vi "loim.vi"() -> ()   [LabVIEW 2015]
panel:
  out "Játékos neve:":string
  out "Nyereménye:":string
  out "Nyereménylista:":i32(listbox)
  out "D válasz":string
  out "C válasz":string
  out "B válasz":string
  out "A válasz":string
  out "Kérdés":string
  in  "Kilépés":bool
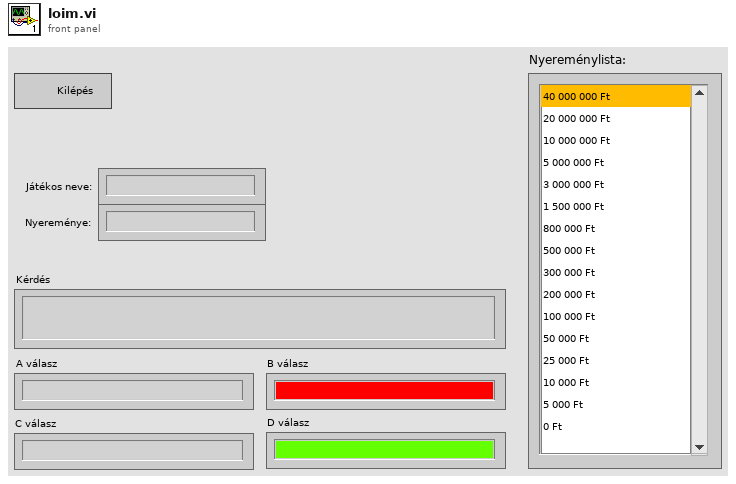
[diagram p1: front panel]
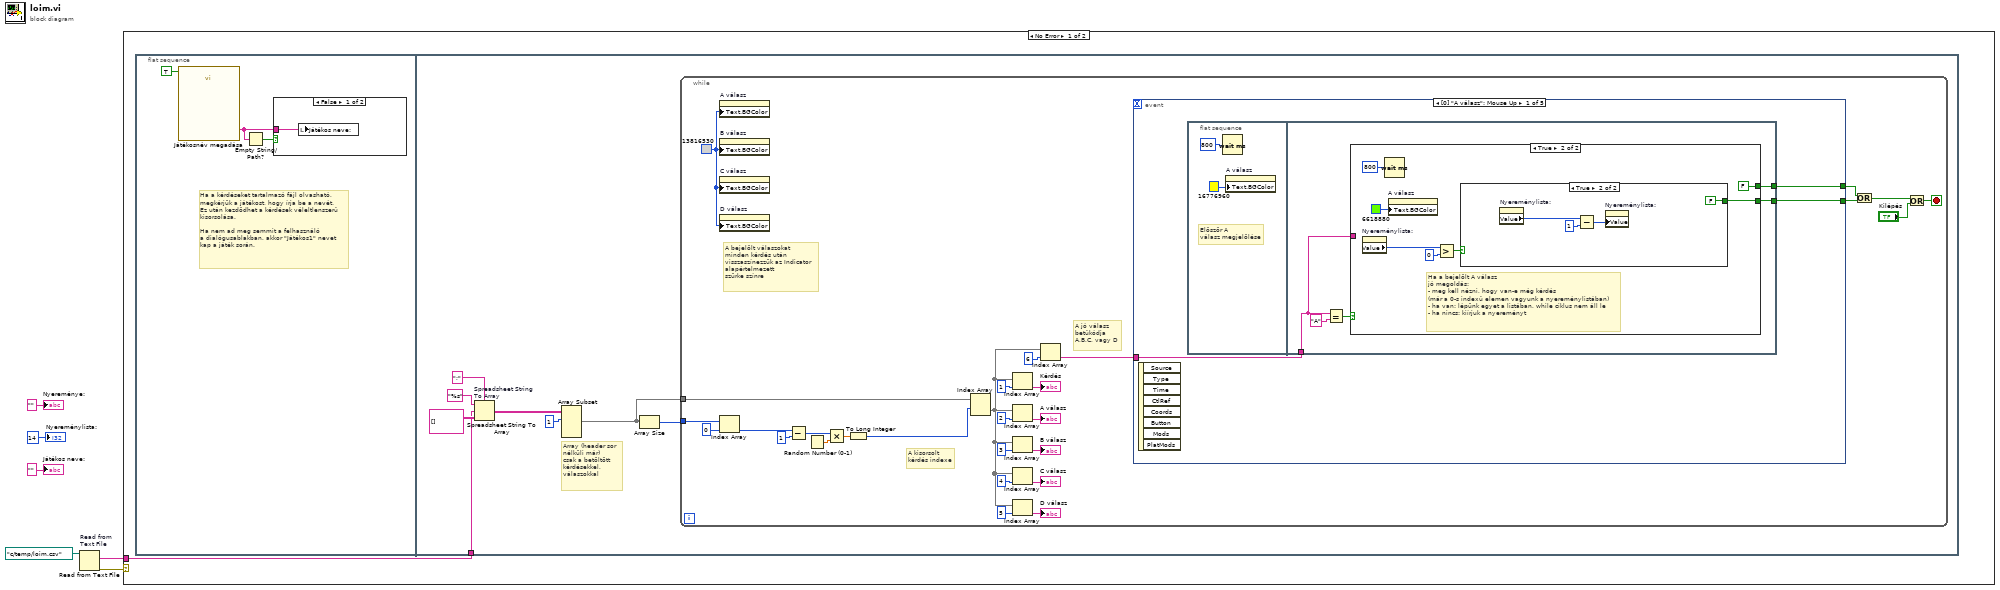
[diagram p0: block diagram]
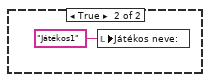
[diagram p2: hidden frame]
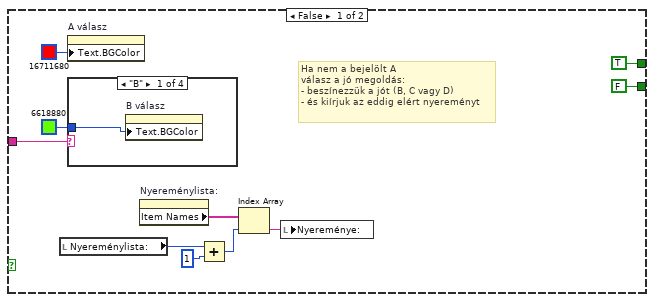
[diagram p3: hidden frame]
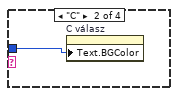
[diagram p4: hidden frame]
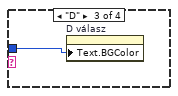
[diagram p5: hidden frame]
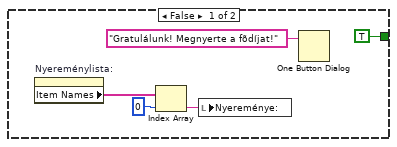
[diagram p7: hidden frame]
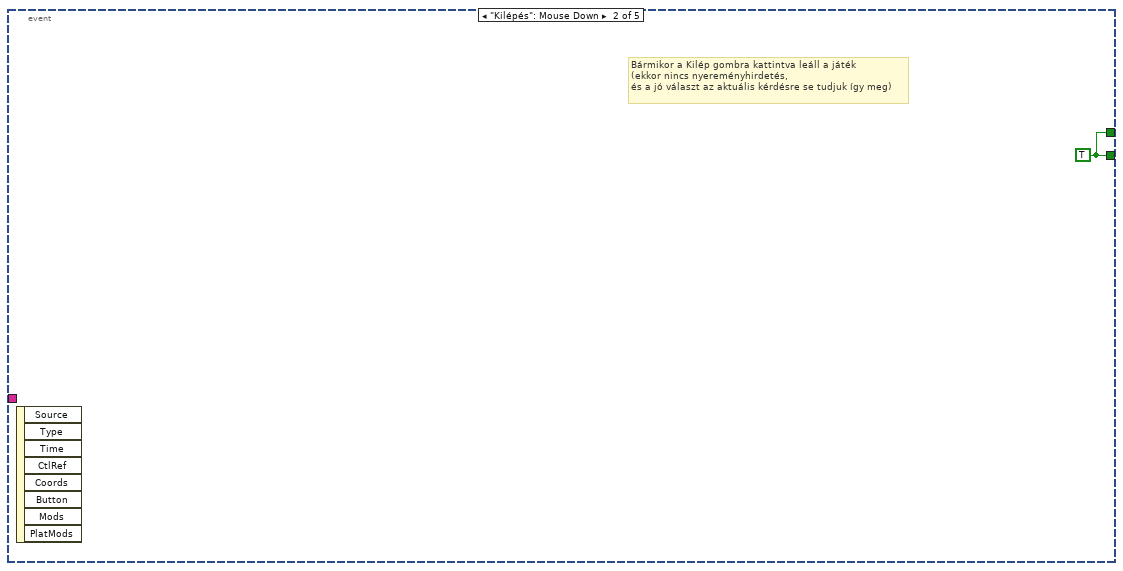
[diagram p8: hidden frame]
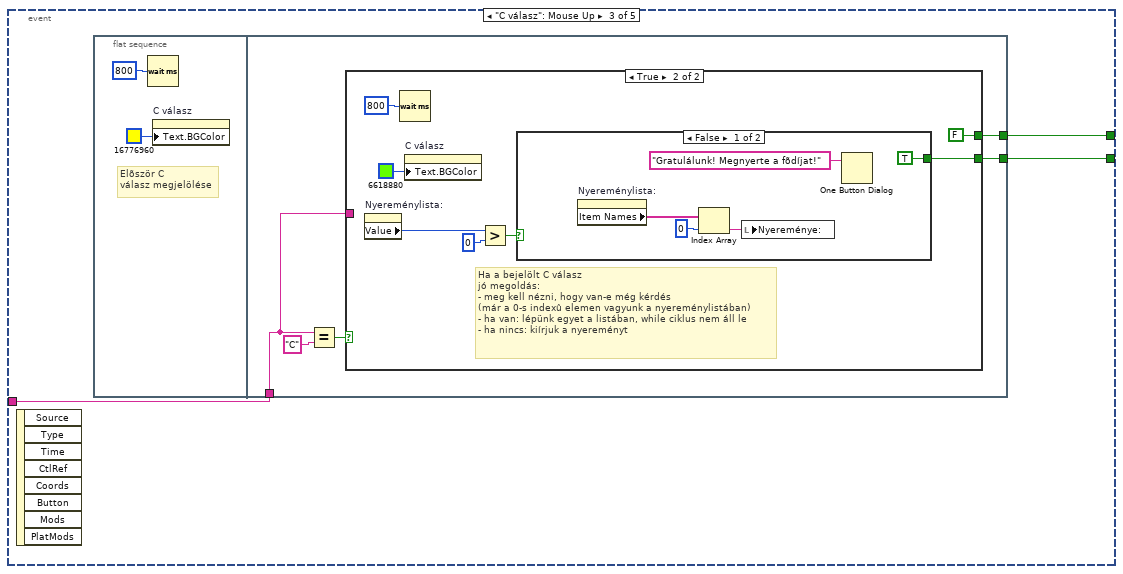
[diagram p9: hidden frame]
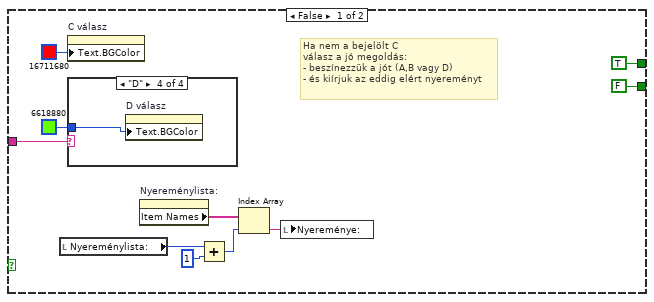
[diagram p10: hidden frame]
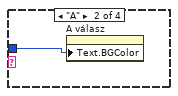
[diagram p12: hidden frame]
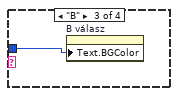
[diagram p13: hidden frame]
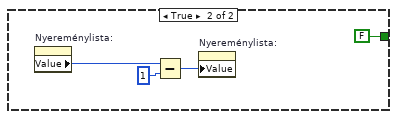
[diagram p14: hidden frame]
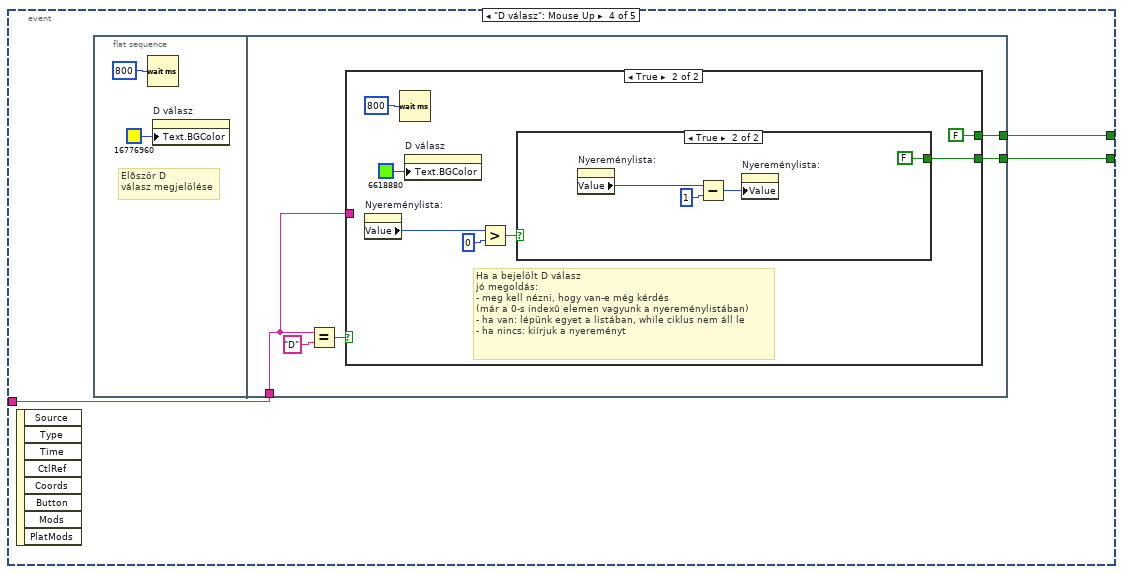
[diagram p15: hidden frame]
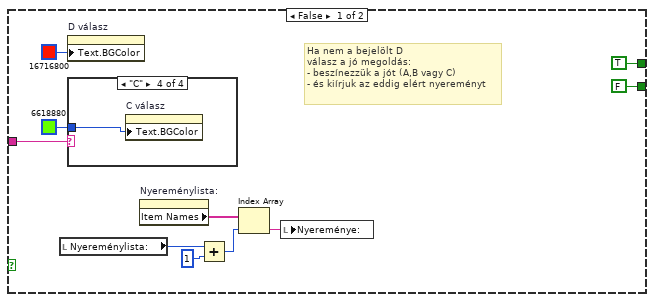
[diagram p16: hidden frame]
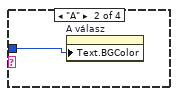
[diagram p18: hidden frame]
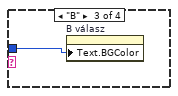
[diagram p19: hidden frame]
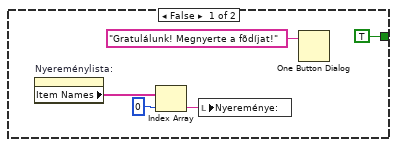
[diagram p20: hidden frame]
diagram:
  n1 = Read from Text File "Read from\nText File"(file (use dialog)=path "c:/temp/loim.csv") -> (text=w1:string, error out=w2:errorcluster)  [unwired: 3 in, 2 out]
  n2 = case shown="No Error" w2 {
    tunnel: w1 -> [w7 _]
    frame No Error {
      n3 = flat-sequence {
        tunnel: w7 -> [w13]
        frame #0 {
          # "Ha a kérdéseket tartalmazó fájl olvasható,\nmegkérjük a játékost, hogy írja be a nevét.\nEz után kezdõdhet a kérdések véleltlenszerû\nkisorsolása.\n\nHa nem ad meg semmit a felhasználó\na dialógusablakban, akkor \"Játékos1\" nevet\nkap a játék során."
          n4 = call "Játékosnév megadása"("Enable"=TRUE) -> ("Adja meg a nevét:"=w8:string)  [unwired: 16 in, 2 out]
          n5 = Empty String/Path?(string/path=w8) -> (empty?=w9:bool)
          n6 = case shown="False" w9 {
            tunnel: w8 -> [w11 _]
            frame False {
              n7 = local write "Játékos neve:"(w11) -> ()
            }
            frame True {
              n8 = local write "Játékos neve:"("Játékos1" ("Játékos neve:")) -> ()
            }
          }
        }
        frame #1 {
          # "Array (header sor\nnélküli már)\ncsak a betöltött\nkérdésekkel,\nválaszokkal"
          n9 = Spreadsheet String To Array "Spreadsheet String\nTo Array"(delimiter (Tab)=";", format string="%s", spreadsheet string=w13, array type (2D Dbl)=string[][] []) -> (array=w17:string[][])
          n10 = Array Subset "Array Subset"(array=w17, index (row)=1 ("index")) -> (w20:string[][])  [unwired: 3 in]
          n11 = Array Size(array=w20) -> (size(s)=w19:i32[])
          n12 = while {
            tunnel: w19 -> [w23]
            tunnel: w20 -> [w22]
            stop <- w21 stop-if-true
            w31 = u32 13816530
            # "A bejelölt válaszokat\nminden kérdés után\nvisszaszínezzük az Indicator\nalapértelmezett\nszürke színre"
            # "A kisorsolt\nkérdés indexe"
            # "A jó válasz\nbetûkódja\nA,B,C, vagy D"
            n13 = property on="A válasz" class="Str"("Text.BGColor"=w31) -> ()  [unwired: 2 in, 2 out]
            n14 = property on="B válasz" class="Str"("Text.BGColor"=w31) -> ()  [unwired: 2 in, 2 out]
            n15 = property on="C válasz" class="Str"("Text.BGColor"=w31) -> ()  [unwired: 2 in, 2 out]
            n16 = property on="D válasz" class="Str"("Text.BGColor"=w31) -> ()  [unwired: 2 in, 2 out]
            n17 = Index Array "Index Array"(array=w23, index=0) -> (element=w27:i32)
            n18 = Subtract(x=w27, y=1) -> (x-y=w26:i32)
            n19 = Random Number (0-1)() -> (number: 0 to 1=w47:dbl)
            n20 = Multiply(x=w26, y=w47) -> (x*y=w46:dbl)
            n21 = To Long Integer(number=w46) -> (32bit integer=w45:i32)
            n22 = Index Array "Index Array"(array=w22, index (row)=w45) -> (element=w38:string[])  [unwired: 1 in]
            n23 = Index Array(array=w38, index=1) -> (element=→"Kérdés":string)
            n24 = Index Array(array=w38, index=2) -> (element=→"A válasz":string)
            n25 = Index Array(array=w38, index=3) -> (element=→"B válasz":string)
            n26 = Index Array(array=w38, index=4) -> (element=→"C válasz":string)
            n27 = Index Array(array=w38, index=5) -> (element=→"D válasz":string)
            n28 = Index Array "Index Array"(array=w38, index=6) -> (element=w32:string)
            n29 = event shown="[0] \"A válasz\": Mouse Up" {
              selector: _ -> [_ _ _ _ _]
              dyn-events: _ -> [_ _ _ _ _]
              timeout: _ -> [_ _ _ _ _]
              tunnel: w32 -> [w51 _ w89 w130 w169]
              tunnel: [w50 w88 w91 w129 w168] -> w30
              tunnel: [w49 w88 w90 w128 w167] -> w28
              event "A válasz": Mouse Up {
                n30 = event-data() -> ()  [unwired: 1 in, 8 out]
                n31 = flat-sequence {
                  tunnel: w51 -> [w55]
                  tunnel: [w56] -> w50
                  tunnel: [w54] -> w49
                  frame #0 {
                    # "Elõször A\nválasz megjelölése"
                    n32 = Wait (ms)(milliseconds to wait=u32 800) -> ()  [unwired: 1 out]
                    n33 = property on="A válasz" class="Str"("Text.BGColor"=u32 16776960) -> ()  [unwired: 2 in, 2 out]
                  }
                  frame #1 {
                    n34 = Equal?(x=w55, y="A") -> (x = y?=w57:bool)
                    n35 = case shown="True" w57 {
                      tunnel: [TRUE FALSE] -> w56
                      tunnel: w55 -> [w62 _]
                      tunnel: [FALSE w72] -> w54
                      frame False {
                        # "Ha nem a bejelölt A\nválasz a jó megoldás:\n- beszínezzük a jót (B, C vagy D)\n- és kiírjuk az eddig elért nyereményt"
                        n36 = local read "Nyereménylista:"() -> (w65:i32)
                        n37 = property on="A válasz" class="Str"("Text.BGColor"=u32 16711680) -> ()  [unwired: 2 in, 2 out]
                        n38 = case shown="\"B\"" w62 {
                          tunnel: u32 6618880 -> [w69 w70 w71 _]
                          frame "B" {
                            n39 = property on="B válasz" class="Str"("Text.BGColor"=w69) -> ()  [unwired: 2 in, 2 out]
                          }
                          frame "C" {
                            n40 = property on="C válasz" class="Str"("Text.BGColor"=w70) -> ()  [unwired: 2 in, 2 out]
                          }
                          frame "D" {
                            n41 = property on="D válasz" class="Str"("Text.BGColor"=w71) -> ()  [unwired: 2 in, 2 out]
                          }
                          frame "", Default {
                          }
                        }
                        n42 = property on="Nyereménylista:" class="LstBox (strict)"() -> ("Item Names"=w66:string[])  [unwired: 2 in, 2 out]
                        n43 = Add(x=w65, y=1) -> (x+y=w63:i32)
                        n44 = Index Array(array=w66, index=w63) -> (element=w59:string)
                        n45 = local write "Nyereménye:"(w59) -> ()
                      }
                      frame True {
                        # "Ha a bejelölt A válasz\njó megoldás:\n- meg kell nézni, hogy van-e még kérdés\n(már a 0-s indexû elemen vagyunk a nyereménylistában)\n- ha van: lépünk egyet a listában, while ciklus nem áll le\n- ha nincs: kiírjuk a nyereményt"
                        n46 = property on="Nyereménylista:" class="LstBox (strict)"() -> ("Value"=w75:i32)  [unwired: 2 in, 2 out]
                        n47 = Wait (ms)(milliseconds to wait=u32 800) -> ()  [unwired: 1 out]
                        n48 = property on="A válasz" class="Str"("Text.BGColor"=u32 6618880) -> ()  [unwired: 2 in, 2 out]
                        n49 = Greater?(x=w75, y=0) -> (0:w73:bool)
                        n50 = case shown="True" w73 {
                          tunnel: [TRUE FALSE] -> w72
                          frame False {
                            n51 = property on="Nyereménylista:" class="LstBox (strict)"() -> ("Item Names"=w80:string[])  [unwired: 2 in, 2 out]
                            n52 = Index Array(array=w80, index=0) -> (element=w79:string)
                            n53 = local write "Nyereménye:"(w79) -> ()
                            n54 = One Button Dialog(message="Gratulálunk! Megnyerte a fõdíjat!") -> ()  [unwired: 1 in, 1 out]
                          }
                          frame True {
                            n55 = property on="Nyereménylista:" class="LstBox (strict)"() -> ("Value"=w85:i32)  [unwired: 2 in, 2 out]
                            n56 = Subtract(x=w85, y=1) -> (x-y=w86:i32)
                            n57 = property on="Nyereménylista:" class="LstBox (strict)"("Value"=w86) -> ()  [unwired: 2 in, 2 out]
                          }
                        }
                      }
                    }
                  }
                }
              }
              event "Kilépés": Mouse Down {
                w88 = TRUE
                # "Bármikor a Kilép gombra kattintva leáll a játék\n(ekkor nincs nyereményhirdetés, \nés a jó választ az aktuális kérdésre se tudjuk így meg)"
                n58 = event-data() -> ()  [unwired: 1 in, 8 out]
              }
              event "C válasz": Mouse Up {
                n59 = event-data() -> ()  [unwired: 1 in, 8 out]
                n60 = flat-sequence {
                  tunnel: [w97] -> w91
                  tunnel: [w96] -> w90
                  tunnel: w89 -> [w95]
                  frame #0 {
                    # "Elõször C\nválasz megjelölése"
                    n61 = Wait (ms)(milliseconds to wait=u32 800) -> ()  [unwired: 1 out]
                    n62 = property on="C válasz" class="Str"("Text.BGColor"=u32 16776960) -> ()  [unwired: 2 in, 2 out]
                  }
                  frame #1 {
                    n63 = Equal?(x=w95, y="C") -> (x = y?=w98:bool)
                    n64 = case shown="True" w98 {
                      tunnel: [TRUE FALSE] -> w97
                      tunnel: [FALSE w112] -> w96
                      tunnel: w95 -> [w107 _]
                      frame False {
                        # "Ha nem a bejelölt C\nválasz a jó megoldás:\n- beszínezzük a jót (A,B vagy D)\n- és kiírjuk az eddig elért nyereményt"
                        n65 = local read "Nyereménylista:"() -> (w105:i32)
                        n66 = property on="C válasz" class="Str"("Text.BGColor"=u32 16711680) -> ()  [unwired: 2 in, 2 out]
                        n67 = case shown="\"D\"" w107 {
                          tunnel: u32 6618880 -> [_ w109 w110 w111]
                          frame "", Default {
                          }
                          frame "A" {
                            n68 = property on="A válasz" class="Str"("Text.BGColor"=w109) -> ()  [unwired: 2 in, 2 out]
                          }
                          frame "B" {
                            n69 = property on="B válasz" class="Str"("Text.BGColor"=w110) -> ()  [unwired: 2 in, 2 out]
                          }
                          frame "D" {
                            n70 = property on="D válasz" class="Str"("Text.BGColor"=w111) -> ()  [unwired: 2 in, 2 out]
                          }
                        }
                        n71 = property on="Nyereménylista:" class="LstBox (strict)"() -> ("Item Names"=w102:string[])  [unwired: 2 in, 2 out]
                        n72 = Add(x=w105, y=1) -> (x+y=w103:i32)
                        n73 = Index Array(array=w102, index=w103) -> (element=w101:string)
                        n74 = local write "Nyereménye:"(w101) -> ()
                      }
                      frame True {
                        # "Ha a bejelölt C válasz\njó megoldás:\n- meg kell nézni, hogy van-e még kérdés\n(már a 0-s indexû elemen vagyunk a nyereménylistában)\n- ha van: lépünk egyet a listában, while ciklus nem áll le\n- ha nincs: kiírjuk a nyereményt"
                        n75 = property on="Nyereménylista:" class="LstBox (strict)"() -> ("Value"=w116:i32)  [unwired: 2 in, 2 out]
                        n76 = Wait (ms)(milliseconds to wait=u32 800) -> ()  [unwired: 1 out]
                        n77 = property on="C válasz" class="Str"("Text.BGColor"=u32 6618880) -> ()  [unwired: 2 in, 2 out]
                        n78 = Greater?(x=w116, y=0) -> (0:w113:bool)
                        n79 = case shown="False" w113 {
                          tunnel: [TRUE FALSE] -> w112
                          frame False {
                            n80 = property on="Nyereménylista:" class="LstBox (strict)"() -> ("Item Names"=w123:string[])  [unwired: 2 in, 2 out]
                            n81 = Index Array(array=w123, index=0) -> (element=w121:string)
                            n82 = local write "Nyereménye:"(w121) -> ()
                            n83 = One Button Dialog(message="Gratulálunk! Megnyerte a fõdíjat!") -> ()  [unwired: 1 in, 1 out]
                          }
                          frame True {
                            n84 = property on="Nyereménylista:" class="LstBox (strict)"() -> ("Value"=w125:i32)  [unwired: 2 in, 2 out]
                            n85 = Subtract(x=w125, y=1) -> (x-y=w126:i32)
                            n86 = property on="Nyereménylista:" class="LstBox (strict)"("Value"=w126) -> ()  [unwired: 2 in, 2 out]
                          }
                        }
                      }
                    }
                  }
                }
              }
              event "D válasz": Mouse Up {
                n87 = event-data() -> ()  [unwired: 1 in, 8 out]
                n88 = flat-sequence {
                  tunnel: w130 -> [w133]
                  tunnel: [w135] -> w129
                  tunnel: [w134] -> w128
                  frame #0 {
                    # "Elõször D\nválasz megjelölése"
                    n89 = Wait (ms)(milliseconds to wait=u32 800) -> ()  [unwired: 1 out]
                    n90 = property on="D válasz" class="Str"("Text.BGColor"=u32 16776960) -> ()  [unwired: 2 in, 2 out]
                  }
                  frame #1 {
                    n91 = Equal?(x=w133, y="D") -> (x = y?=w137:bool)
                    n92 = case shown="True" w137 {
                      tunnel: [TRUE FALSE] -> w135
                      tunnel: [FALSE w151] -> w134
                      tunnel: w133 -> [w146 _]
                      frame False {
                        # "Ha nem a bejelölt D\nválasz a jó megoldás:\n- beszínezzük a jót (A,B vagy C)\n- és kiírjuk az eddig elért nyereményt"
                        n93 = local read "Nyereménylista:"() -> (w140:i32)
                        n94 = property on="D válasz" class="Str"("Text.BGColor"=u32 16716800) -> ()  [unwired: 2 in, 2 out]
                        n95 = case shown="\"C\"" w146 {
                          tunnel: u32 6618880 -> [_ w148 w149 w150]
                          frame "", Default {
                          }
                          frame "A" {
                            n96 = property on="A válasz" class="Str"("Text.BGColor"=w148) -> ()  [unwired: 2 in, 2 out]
                          }
                          frame "B" {
                            n97 = property on="B válasz" class="Str"("Text.BGColor"=w149) -> ()  [unwired: 2 in, 2 out]
                          }
                          frame "C" {
                            n98 = property on="C válasz" class="Str"("Text.BGColor"=w150) -> ()  [unwired: 2 in, 2 out]
                          }
                        }
                        n99 = property on="Nyereménylista:" class="LstBox (strict)"() -> ("Item Names"=w141:string[])  [unwired: 2 in, 2 out]
                        n100 = Add(x=w140, y=1) -> (x+y=w138:i32)
                        n101 = Index Array(array=w141, index=w138) -> (element=w142:string)
                        n102 = local write "Nyereménye:"(w142) -> ()
                      }
                      frame True {
                        # "Ha a bejelölt D válasz\njó megoldás:\n- meg kell nézni, hogy van-e még kérdés\n(már a 0-s indexû elemen vagyunk a nyereménylistában)\n- ha van: lépünk egyet a listában, while ciklus nem áll le\n- ha nincs: kiírjuk a nyereményt"
                        n103 = property on="Nyereménylista:" class="LstBox (strict)"() -> ("Value"=w155:i32)  [unwired: 2 in, 2 out]
                        n104 = Wait (ms)(milliseconds to wait=u32 800) -> ()  [unwired: 1 out]
                        n105 = property on="D válasz" class="Str"("Text.BGColor"=u32 6618880) -> ()  [unwired: 2 in, 2 out]
                        n106 = Greater?(x=w155, y=0) -> (0:w152:bool)
                        n107 = case shown="True" w152 {
                          tunnel: [TRUE FALSE] -> w151
                          frame False {
                            n108 = property on="Nyereménylista:" class="LstBox (strict)"() -> ("Item Names"=w160:string[])  [unwired: 2 in, 2 out]
                            n109 = Index Array(array=w160, index=0) -> (element=w159:string)
                            n110 = local write "Nyereménye:"(w159) -> ()
                            n111 = One Button Dialog(message="Gratulálunk! Megnyerte a fõdíjat!") -> ()  [unwired: 1 in, 1 out]
                          }
                          frame True {
                            n112 = property on="Nyereménylista:" class="LstBox (strict)"() -> ("Value"=w165:i32)  [unwired: 2 in, 2 out]
                            n113 = Subtract(x=w165, y=1) -> (x-y=w163:i32)
                            n114 = property on="Nyereménylista:" class="LstBox (strict)"("Value"=w163) -> ()  [unwired: 2 in, 2 out]
                          }
                        }
                      }
                    }
                  }
                }
              }
              event "B válasz": Mouse Up {
                n115 = event-data() -> ()  [unwired: 1 in, 8 out]
                n116 = flat-sequence {
                  tunnel: w169 -> [w174]
                  tunnel: [w173] -> w168
                  tunnel: [w172] -> w167
                  frame #0 {
                    # "Elõször B\nválasz megjelölése"
                    n117 = Wait (ms)(milliseconds to wait=u32 800) -> ()  [unwired: 1 out]
                    n118 = property on="B válasz" class="Str"("Text.BGColor"=u32 16776960) -> ()  [unwired: 2 in, 2 out]
                  }
                  frame #1 {
                    n119 = Equal?(x=w174, y="B") -> (x = y?=w175:bool)
                    n120 = case shown="True" w175 {
                      tunnel: w174 -> [w186 _]
                      tunnel: [TRUE FALSE] -> w173
                      tunnel: [FALSE w190] -> w172
                      frame False {
                        # "Ha nem a bejelölt B\nválasz a jó megoldás:\n- beszínezzük a jót (A,C vagy D)\n- és kiírjuk az eddig elért nyereményt"
                        n121 = local read "Nyereménylista:"() -> (w182:i32)
                        n122 = property on="B válasz" class="Str"("Text.BGColor"=u32 16711680) -> ()  [unwired: 2 in, 2 out]
                        n123 = case shown="\"A\"" w186 {
                          tunnel: u32 6618880 -> [_ w187 w188 w189]
                          frame "", Default {
                          }
                          frame "D" {
                            n124 = property on="D válasz" class="Str"("Text.BGColor"=w187) -> ()  [unwired: 2 in, 2 out]
                          }
                          frame "C" {
                            n125 = property on="C válasz" class="Str"("Text.BGColor"=w188) -> ()  [unwired: 2 in, 2 out]
                          }
                          frame "A" {
                            n126 = property on="A válasz" class="Str"("Text.BGColor"=w189) -> ()  [unwired: 2 in, 2 out]
                          }
                        }
                        n127 = property on="Nyereménylista:" class="LstBox (strict)"() -> ("Item Names"=w180:string[])  [unwired: 2 in, 2 out]
                        n128 = Add(x=w182, y=1) -> (x+y=w183:i32)
                        n129 = Index Array(array=w180, index=w183) -> (element=w179:string)
                        n130 = local write "Nyereménye:"(w179) -> ()
                      }
                      frame True {
                        # "Ha a bejelölt B válasz\njó megoldás:\n- meg kell nézni, hogy van-e még kérdés\n(már a 0-s indexû elemen vagyunk a nyereménylistában)\n- ha van: lépünk egyet a listában, while ciklus nem áll le\n- ha nincs: kiírjuk a nyereményt"
                        n131 = property on="Nyereménylista:" class="LstBox (strict)"() -> ("Value"=w194:i32)  [unwired: 2 in, 2 out]
                        n132 = Wait (ms)(milliseconds to wait=u32 800) -> ()  [unwired: 1 out]
                        n133 = property on="B válasz" class="Str"("Text.BGColor"=u32 6618880) -> ()  [unwired: 2 in, 2 out]
                        n134 = Greater?(x=w194, y=0) -> (0:w192:bool)
                        n135 = case shown="False" w192 {
                          tunnel: [TRUE FALSE] -> w190
                          frame False {
                            n136 = property on="Nyereménylista:" class="LstBox (strict)"() -> ("Item Names"=w200:string[])  [unwired: 2 in, 2 out]
                            n137 = Index Array "Index Array"(array=w200, index=0) -> (element=w198:string)
                            n138 = One Button Dialog(message="Gratulálunk! Megnyerte a fõdíjat!") -> ()  [unwired: 1 in, 1 out]
                            n139 = local write "Nyereménye:"(w198) -> ()
                          }
                          frame True {
                            n140 = property on="Nyereménylista:" class="LstBox (strict)"() -> ("Value"=w204:i32)  [unwired: 2 in, 2 out]
                            n141 = Subtract(x=w204, y=1) -> (x-y=w205:i32)
                            n142 = property on="Nyereménylista:" class="LstBox (strict)"("Value"=w205) -> ()  [unwired: 2 in, 2 out]
                          }
                        }
                      }
                    }
                  }
                }
              }
            }
            n143 = Or(x=w30, y=w28) -> (x .or. y?=w29:bool)
            n144 = Or(x=w29, y="Kilépés") -> (x .or. y?=w21:bool)
          }
        }
      }
    }
    frame Error {
      (unwired) "Kilépés" ("button name (\"OK\")")
      n145 = One Button Dialog(message="Hiba történt a fájl betöltésekor! \nEllenõrizze, hogy a kérdéseket tartalmazó fájl elérhetõ-e a\nC:\\Temp\\loim.csv helyen!" ("string")) -> ()  [unwired: 1 in, 1 out]
    }
  }
  "Nyereménylista:" <- 14 ("Nyereménylista:")
  "Nyereménye:" <- "" ("Nyeremény:")
  "Játékos neve:" <- "" ("Játékos neve:")
